vi "EVM_Sweep_Only_R_S_CMP180_SpecialCASE.vi"() -> ()   [LabVIEW 2023, in "EVM.lvlib"]
uses:
  lib/CTL/LitePoint_EVM_SG.ctl
  lib/CTL/LitePoint_EVM_SA.ctl
  EVM.lvlib
  lib/LitePoints/LitePoints.lvlib
  lib/FTDI/JIO/CLC_JIO_FTDI.lvlib
  lib/R_S/R_S.lvlib
panel:
  out "ReceivedPower":dbl format="%#.3g"
  out "Best EVM ALL":dbl
  out "PST(sec)":dbl
  out "Best EVM":dbl
  out "error out":errorcluster
  in  "Power res":i32=2
  in  "Stop Power":i32
  in  "Start Power":i32=-40
  in  "BFIC_ele_stop":i32=12
  in  "BFIC_ele_res":i32=4
  in  "BFIC_ele_start":i32
  in  "BFIC_com_stop":i32=12
  in  "BFIC_com_res":i32=4
  in  "BFIC_com_start":i32
  in  "UD_att_stop":i32=120
  in  "UD_att_res":i32=8
  in  "UD_att_start":i32
  out "UD_att":i32=255
  out "BFIC_com_step":i32=15
  out "BFIC_ele_step":i32=15
  out "SG Power":i32=-10
  in  "TRXmode":u16(ring)=1 items=["Tx"=1, "Rx"=2]
  in  "Polarity":u16(ring) items=["H", "V"]
  out "floder Exist?":bool=TRUE
  in  "Waiting \nTime(ms)":u32=1
  in  "FileNote":string="test16_wayne_MCS11"
  in  "SG":refnum<visa-resource-name>="TCPIP0::192.168.200.50::hislip0::INSTR"
  in  "SA":refnum<visa-resource-name>="TCPIP0::192.168.200.50::hislip0::INSTR"
  out "Spectrum Data":cluster{"X":dbl, "Y":dbl}[](graph)
  # "TMYTEK_CLC_JIO_R&S_EVM_CMP180_StartMaxPOWER"
  # "`"
  # "12"
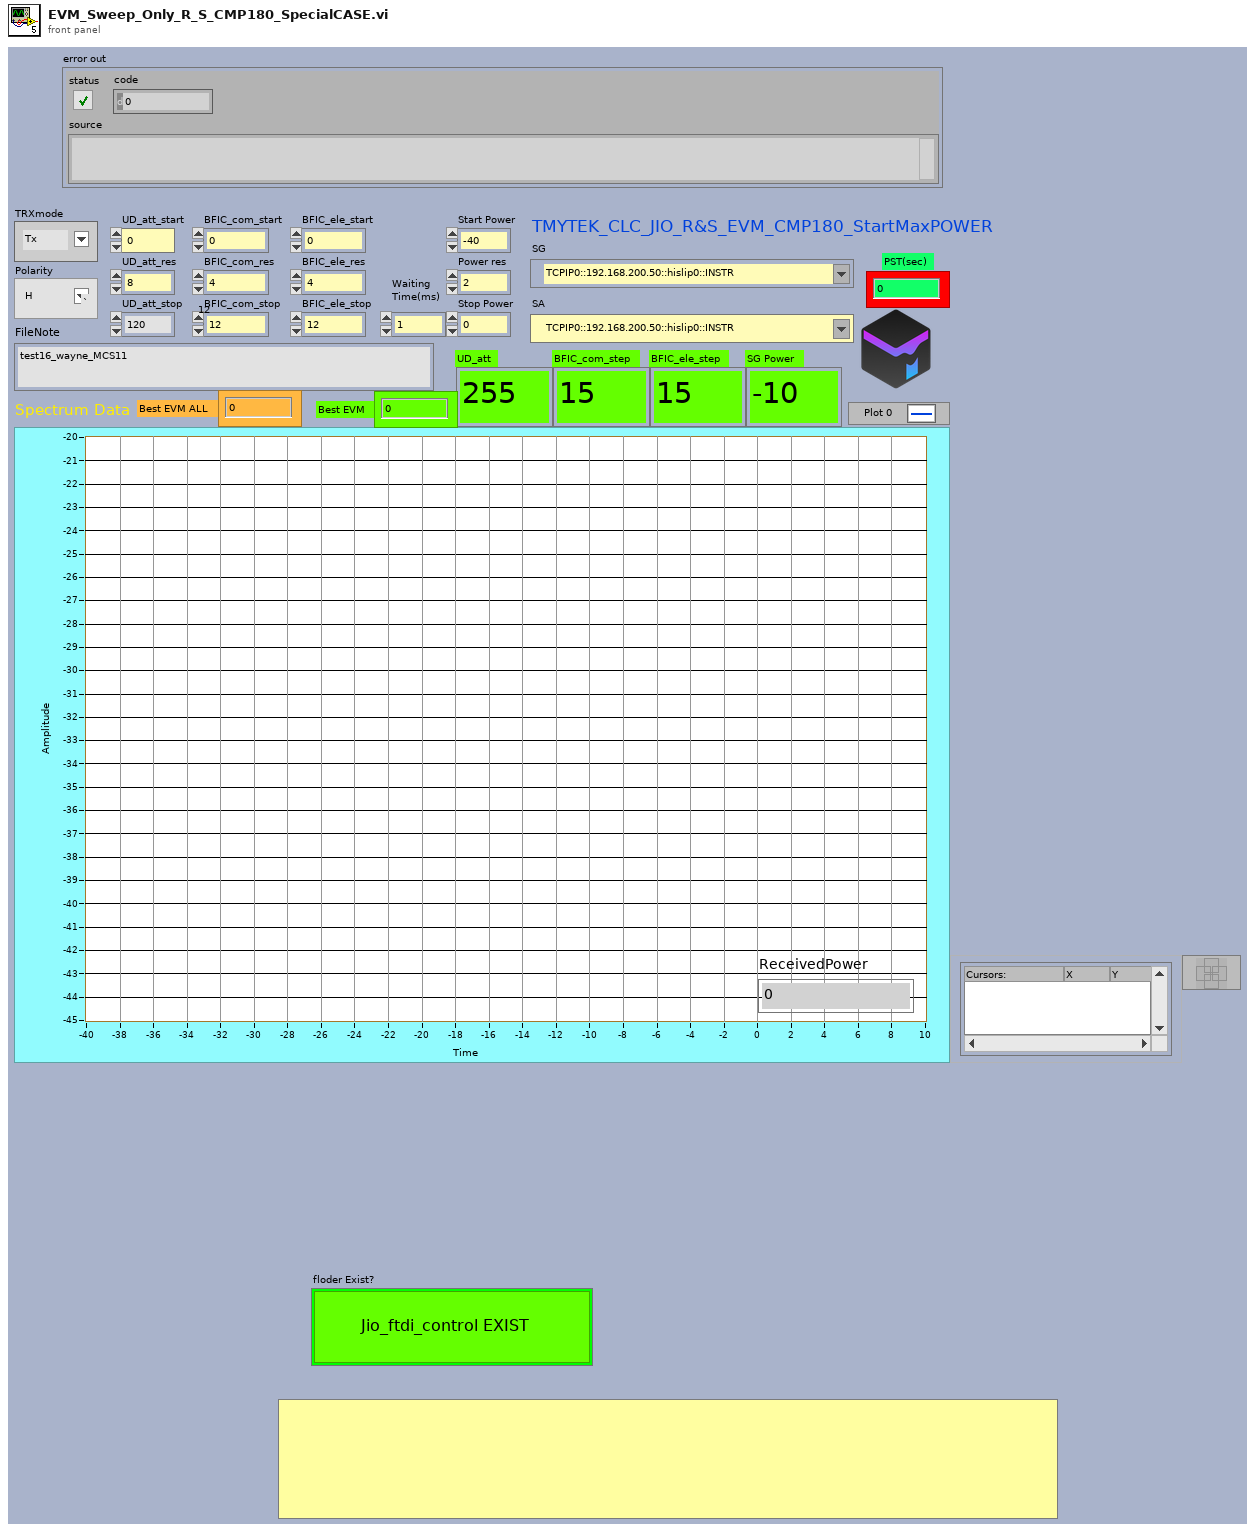
[diagram p1: front panel]
types:
  T1 = typedef "LitePoint_EVM_SG.ctl" = enum16{"Init", "Close", "set_SG", "AdjustLevel", "byPass", "RF_ON", "RF_OFF"}
  T2 = typedef "LitePoint_EVM_SA.ctl" = enum16{"Init", "Close", "set_SA", "get_EVM", "byPass", "getPower"}
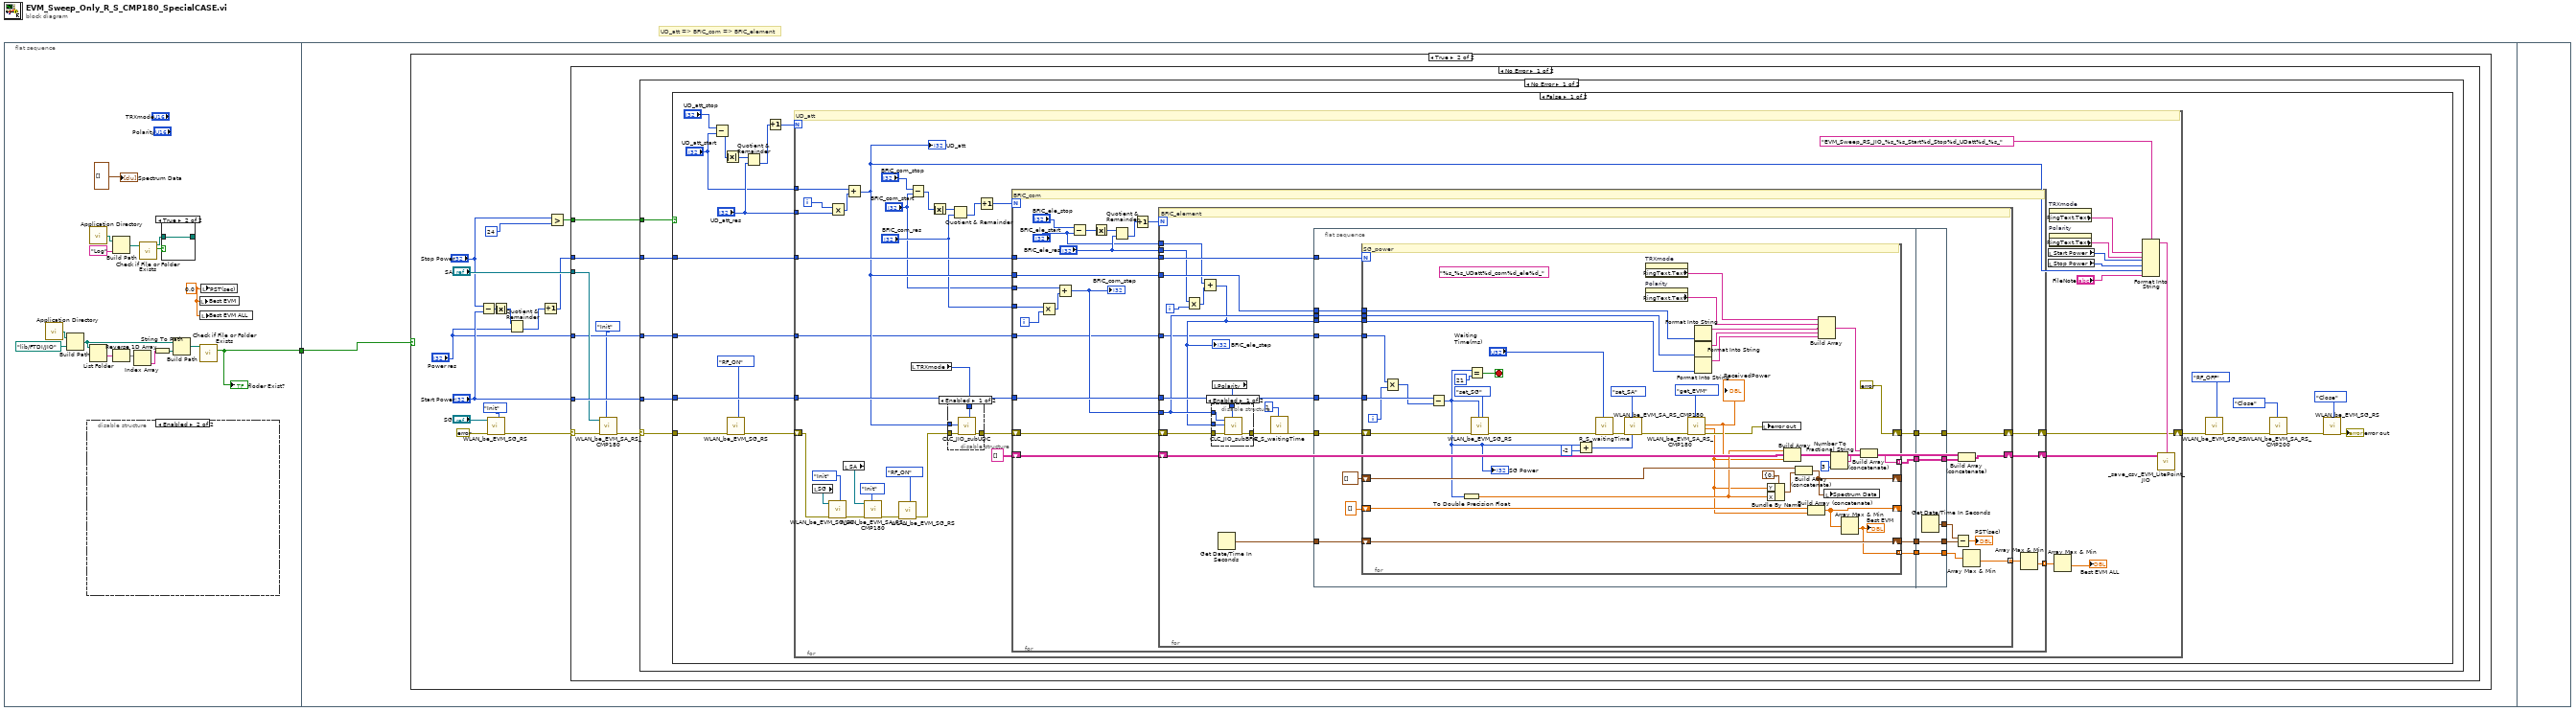
[diagram p0: block diagram]
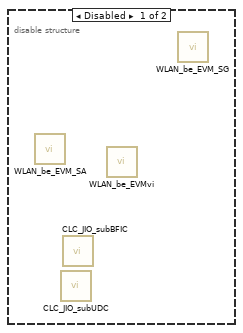
[diagram p2: hidden frame]
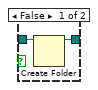
[diagram p3: hidden frame]
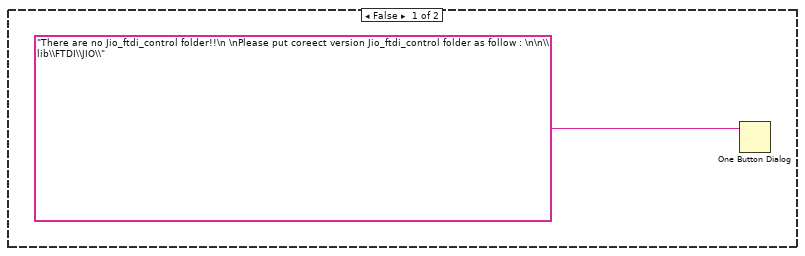
[diagram p4: hidden frame]
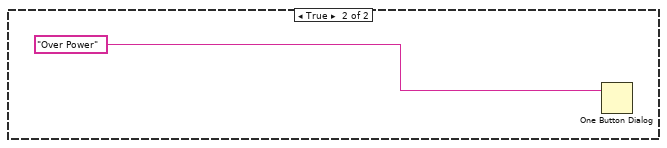
[diagram p7: hidden frame]
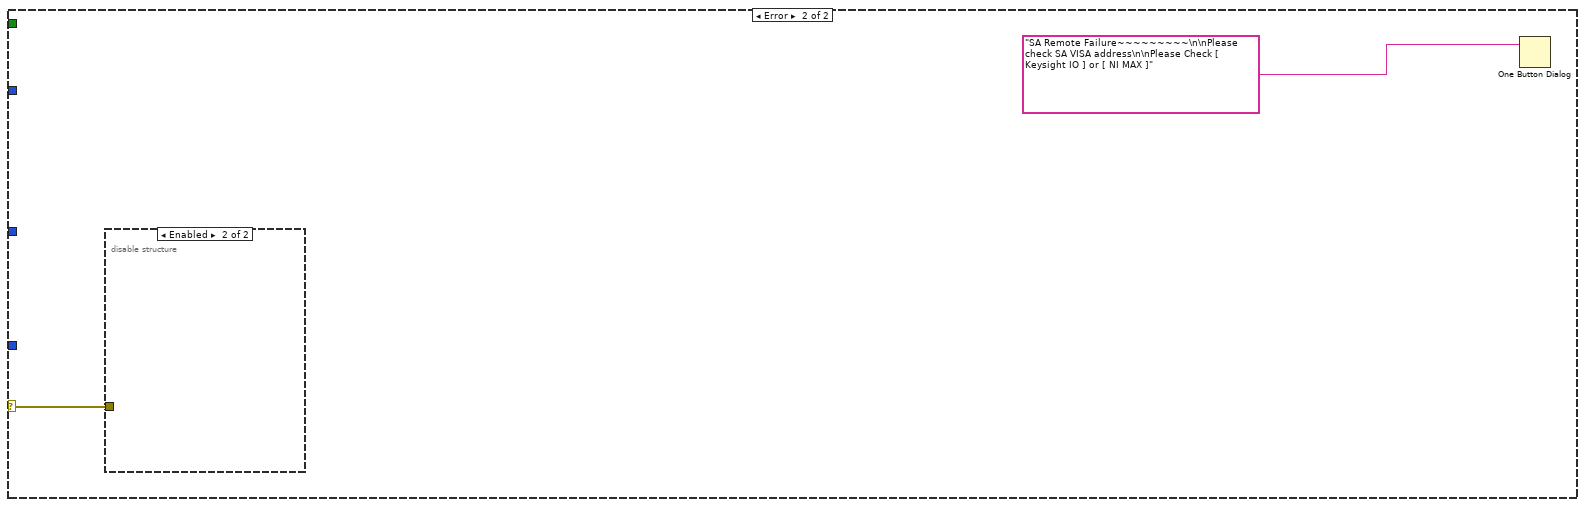
[diagram p8: hidden frame]
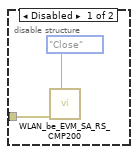
[diagram p9: hidden frame]
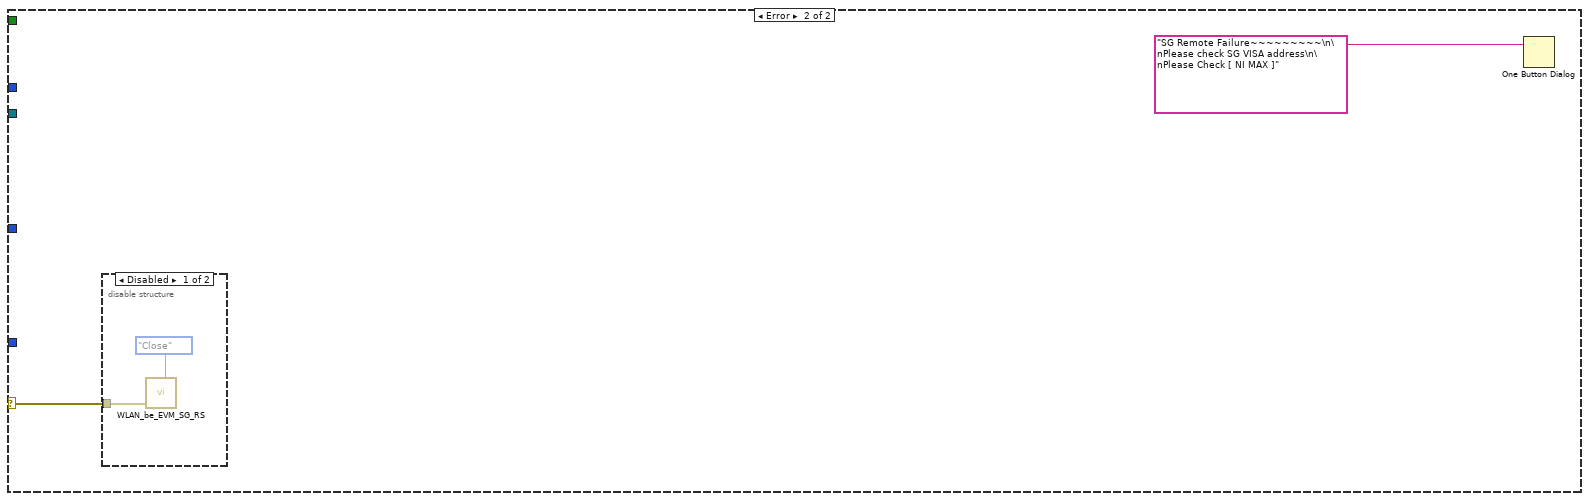
[diagram p10: hidden frame]
diagram:
  # "UD_att => BFIC_com => BFIC_element"
  n1 = flat-sequence {
    tunnel: [w3] -> w1
    tunnel: w1 -> [w21]
    frame #0 {
      w2 = 0.0 ("PST(sec)")
      n2 = call <vilib>:"Application Directory.vi"() -> ("Application Directory"=w9:path)
      n3 = Build Path(base path=w9, name or relative path=path "lib/FTDI/JIO") -> (appended path=w10:path)
      n4 = disable-structure shown="Enabled" {
        frame Disabled {
          n5 = call "WLAN_be_EVM_SA.vi"() -> ()  [unwired: 8 in, 4 out]
          n6 = call "CLC_JIO_subUDC.vi"() -> ()  [unwired: 10 in, 2 out]
          n7 = call "CLC_JIO_subBFIC.vi"() -> ()  [unwired: 10 in, 2 out]
          n8 = call "WLAN_be_EVMvi.vi"() -> ()  [unwired: 8 in, 4 out]
          n9 = call "WLAN_be_EVM_SG.vi"() -> ()  [unwired: 10 in, 2 out]
        }
        frame Enabled {
        }
      }
      n10 = call <vilib>:"Application Directory.vi"() -> ("Application Directory"=w16:path)
      n11 = List Folder(path=w10) -> (folder names=w5:string[])  [unwired: 3 in, 3 out]
      n12 = Reverse 1D Array(array=w5) -> (reversed array=w6:string[])
      n13 = Build Path(base path=w16, name or relative path="Log") -> (appended path=w13:path)
      n14 = Index Array(array=w6) -> (element=w7:string)  [unwired: 1 in]
      n15 = call <vilib>:"Check if File or Folder Exists.vi"("path"=w13) -> ("file or folder exists?"=w15:bool, "dup path"=w14:path)  [unwired: 8 in, 1 out]
      n16 = String To Path(string=w7) -> (path=w8:path)
      n17 = case shown="True" w15 {
        tunnel: w14 -> [w19 w20]
        tunnel: [w18 w20] -> _
        frame False {
          n18 = Create Folder(path (use dialog)=w19) -> (created path=w18:path)  [unwired: 2 in, 2 out]
        }
        frame True {
        }
      }
      n19 = Build Path(base path=w10, name or relative path=w8) -> (appended path=w11:path)
      n20 = local write "Best EVM"(w2) -> ()
      n21 = local write "Best EVM ALL"(w2) -> ()
      n22 = call <vilib>:"Check if File or Folder Exists.vi"("path"=w11) -> ("file or folder exists?"=w3:bool)  [unwired: 8 in, 2 out]
      "floder Exist?" <- w3
      n23 = local write "PST(sec)"(w2) -> ()
      "Spectrum Data" <- cluster{"X":dbl, "Y":dbl}[] [] ("XY Graph")
    }
    frame #1 {
      n24 = case shown="True" w21 {
        frame False {
          n25 = One Button Dialog(message="There are no Jio_ftdi_control folder!!\n \nPlease put coreect version Jio_ftdi_control folder as follow : \n\n\\lib\\FTDI\\JIO\\") -> ()  [unwired: 1 in, 1 out]
        }
        frame True {
          n26 = Subtract(x="Stop Power", y="Start Power") -> (x-y=w27:i32)
          n27 = call "WLAN_be_EVM_SG_RS.vi"("Function_SG"=LitePoint_EVM_SG."Init", "error in"=errorcluster {"status"=FALSE, "code"=0, "source"=""} ("error in (no error)"), "VISA IN"="SG") -> ("error out"=w29:errorcluster)  [unwired: 7 in, 1 out]
          n28 = Absolute Value(x=w27) -> (abs(x)=w23:i32)
          n29 = Quotient & Remainder(x=w23, y="Power res") -> (floor(x/y)=w26:i32)  [unwired: 1 out]
          n30 = Increment(x=w26) -> (x+1=w33:i32)
          n31 = Greater?(x="Stop Power", y=24) -> (0:w35:bool)
          n32 = case shown="No Error" w29 {
            selector: w29 -> [w41 w237]
            tunnel: "SA" -> [w39 _]
            tunnel: w35 -> [w44 _]
            tunnel: "Start Power" -> [w43 _]
            tunnel: w33 -> [w42 _]
            tunnel: "Power res" -> [w38 _]
            frame No Error {
              n33 = call "WLAN_be_EVM_SA_RS_CMP180.vi"("Function"=LitePoint_EVM_SA."Init", "error in"=w41, "VISA IN"=w39) -> ("error out"=w40:errorcluster)  [unwired: 4 in, 4 out]
              n34 = case shown="No Error" w40 {
                selector: w40 -> [w46 w233]
                tunnel: w44 -> [w49 _]
                tunnel: w43 -> [w48 _]
                tunnel: w42 -> [w47 _]
                tunnel: w38 -> [w45 _]
                frame No Error {
                  n35 = case shown="False" w49 {
                    tunnel: w48 -> [w68 _]
                    tunnel: w46 -> [w67 _]
                    tunnel: w47 -> [w69 _]
                    tunnel: w45 -> [w55 _]
                    frame False {
                      n36 = Subtract(x="UD_att_stop", y="UD_att_start") -> (x-y=w62:i32)
                      n37 = Absolute Value(x=w62) -> (abs(x)=w59:i32)
                      n38 = call "WLAN_be_EVM_SG_RS.vi"("Function_SG"=LitePoint_EVM_SG."RF_ON", "error in"=w67) -> ("error out"=w65:errorcluster)  [unwired: 8 in, 1 out]
                      n39 = Quotient & Remainder(x=w59, y="UD_att_res") -> (floor(x/y)=w60:i32)  [unwired: 1 out]
                      n40 = Increment(x=w60) -> (x+1=w56:i32)
                      n41 = for {
                        N: w56 -> [_]
                        tunnel: w69 -> [w107]
                        tunnel: w68 -> [w106]
                        shift-right: [w94] -> w64
                        shift-left: w65 -> [w79]
                        tunnel: "UD_att_res" -> [w91]
                        tunnel: "UD_att_start" -> [w90]
                        tunnel: w55 -> [w81]
                        i -> [w93]
                        # "UD_att"
                        n42 = local read "SG"() -> (w76:refnum<visa-resource-name>)
                        n43 = call "WLAN_be_EVM_SG_RS.vi"("Function_SG"=LitePoint_EVM_SG."Init", "error in"=w79, "VISA IN"=w76) -> ("error out"=w77:errorcluster)  [unwired: 7 in, 1 out]
                        n44 = Multiply(x=w93, y=w91) -> (x*y=w92:i32)
                        n45 = local read "SA"() -> (w75:refnum<visa-resource-name>)
                        n46 = Add(x=w90, y=w92) -> (x+y=w89:i32)
                        "UD_att" <- w89
                        n47 = call "WLAN_be_EVM_SA_RS_CMP180.vi"("Function"=LitePoint_EVM_SA."Init", "error in"=w77, "VISA IN"=w75) -> ("error out"=w73:errorcluster)  [unwired: 4 in, 4 out]
                        n48 = call "WLAN_be_EVM_SG_RS.vi"("Function_SG"=LitePoint_EVM_SG."RF_ON", "error in"=w73) -> ("error out"=w72:errorcluster)  [unwired: 8 in, 1 out]
                        n49 = Subtract(x="BFIC_com_stop", y="BFIC_com_start") -> (x-y=w88:i32)
                        n50 = local read "TRXmode"() -> (w103:u16)
                        n51 = Absolute Value(x=w88) -> (abs(x)=w87:i32)
                        n52 = disable-structure shown="Enabled" {
                          disable-tunnel: [w111 w112] -> w105
                          disable-tunnel: w72 -> [w110 w112]
                          disable-tunnel: w103 -> [w109 _]
                          disable-tunnel: w89 -> [w108 _]
                          frame Enabled {
                            n53 = call "CLC_JIO_subUDC.vi"("Mode"=w109, "error in"=w110, "ud att"=w108) -> ("error out"=w111:errorcluster)  [unwired: 7 in, 1 out]
                          }
                          frame Disabled {
                          }
                        }
                        n54 = Quotient & Remainder(x=w87, y="BFIC_com_res") -> (floor(x/y)=w83:i32)  [unwired: 1 out]
                        n55 = Increment(x=w83) -> (x+1=w82:i32)
                        n56 = for {
                          N: w82 -> [_]
                          tunnel: w107 -> [w134]
                          tunnel: w106 -> [w133]
                          shift-right: [w130] -> w104
                          shift-left: string[][] [] -> [w131]
                          tunnel: w89 -> [w129]
                          shift-right: [w128] -> w94
                          shift-left: w105 -> [w132]
                          tunnel: "BFIC_com_res" -> [w124]
                          tunnel: "BFIC_com_start" -> [w123]
                          tunnel: w81 -> [w115]
                          tunnel: [w113] -> w71 mode=indexing
                          i -> [w126]
                          # "BFIC_com"
                          n57 = Multiply(x=w124, y=w126) -> (x*y=w127:i32)
                          n58 = Add(x=w123, y=w127) -> (x+y=w125:i32)
                          "BFIC_com_step" <- w125
                          n59 = Subtract(x="BFIC_ele_stop", y="BFIC_ele_start") -> (x-y=w121:i32)
                          n60 = Absolute Value(x=w121) -> (abs(x)=w122:i32)
                          n61 = Quotient & Remainder(x=w122, y="BFIC_ele_res") -> (floor(x/y)=w119:i32)  [unwired: 1 out]
                          n62 = Increment(x=w119) -> (x+1=w116:i32)
                          n63 = for {
                            N: w116 -> [_]
                            tunnel: w134 -> [w163]
                            tunnel: w133 -> [w162]
                            shift-right: [w160] -> w130
                            shift-left: w131 -> [w159]
                            tunnel: w125 -> [w154]
                            tunnel: w129 -> [w155]
                            shift-right: [w138] -> w128
                            shift-left: w132 -> [w158]
                            tunnel: "BFIC_ele_res" -> [w149]
                            tunnel: "BFIC_ele_start" -> [w148]
                            tunnel: w115 -> [w147]
                            tunnel: [w135] -> w114 mode=indexing
                            i -> [w150]
                            # "BFIC_element"
                            n64 = Multiply(x=w149, y=w150) -> (x*y=w152:i32)
                            n65 = Add(x=w148, y=w152) -> (x+y=w151:i32)
                            "BFIC_ele_step" <- w151
                            n66 = local read "Polarity"() -> (w153:u16)
                            n67 = disable-structure shown="Enabled" {
                              disable-tunnel: w158 -> [w230 w231]
                              disable-tunnel: [w229 w231] -> w157
                              disable-tunnel: w151 -> [w228 _]
                              disable-tunnel: w154 -> [w227 _]
                              disable-tunnel: w153 -> [w226 _]
                              frame Enabled {
                                n68 = call "CLC_JIO_subBFIC.vi"("pol"=w226, "error in"=w230, "ele"=w228, "com"=w227) -> ("error out"=w229:errorcluster)  [unwired: 6 in, 1 out]
                              }
                              frame Disabled {
                              }
                            }
                            n69 = Get Date/Time In Seconds() -> (seconds since 1Jan1904=w145:timestamp)
                            n70 = call "R_S_waitingTime.vi"("Waiting Time(ms)"=u32 1, "error in"=w157) -> ("error out"=w146:errorcluster)  [unwired: 9 in]
                            n71 = flat-sequence {
                              tunnel: w163 -> [w177]
                              tunnel: w162 -> [w175]
                              tunnel: w155 -> [w173]
                              tunnel: w154 -> [w172]
                              tunnel: w151 -> [w170]
                              tunnel: w147 -> [w169]
                              tunnel: w146 -> [w168]
                              tunnel: w145 -> [w166]
                              tunnel: [w174] -> w143
                              tunnel: [w171] -> w142
                              tunnel: [w165] -> w141
                              tunnel: [w164] -> w137
                              tunnel: [w223] -> w144
                              tunnel: [w224] -> w138
                              tunnel: [w225] -> w161
                              tunnel: w143 -> [w225]
                              tunnel: w142 -> [w224]
                              tunnel: w141 -> [w223]
                              tunnel: [w222] -> w140
                              tunnel: [w221] -> w136
                              tunnel: w137 -> [w221]
                              frame #0 {
                                n72 = for {
                                N: w177 -> [_]
                                tunnel: w175 -> [w220]
                                shift-right: [errorcluster {"status"=FALSE, "code"=0, "source"=""} ("error out")] -> w171
                                shift-left: w168 -> [w212]
                                shift-right: [w214] -> _
                                shift-left: cluster{"X":dbl, "Y":dbl}[] [] ("XY Graph") -> [w216]
                                tunnel: [w204] -> w174 mode=indexing
                                tunnel: w173 -> [w201]
                                tunnel: w170 -> [w199]
                                tunnel: w172 -> [w200]
                                tunnel: w169 -> [w193]
                                shift-right: [w181] -> _
                                shift-left: dbl[] [] -> [w183]
                                shift-right: [w180] -> w165
                                shift-left: w166 -> [w180]
                                tunnel: [w178] -> w164 mode=indexing
                                i -> [w194]
                                stop <- w218 stop-if-true
                                (unwired) "%s_%s_UDatt%d_com%d_ele%d_" ("format string")
                                # "SG_power"
                                n73 = Multiply(x=w193, y=w194) -> (x*y=w192:i32)
                                n74 = Subtract(x=w220, y=w192) -> (x-y=w186:i32)
                                "SG Power" <- w186
                                n75 = To Double Precision Float(number=w186) -> (double precision float=w213:dbl)
                                n76 = Equal?(x=w186, y=21) -> (x = y?=w218:bool)
                                n77 = call "WLAN_be_EVM_SG_RS.vi"("Function_SG"=LitePoint_EVM_SG."set_SG", "setPower"=w186, "error in"=w212) -> ("error out"=w190:errorcluster)  [unwired: 7 in, 1 out]
                                n78 = Add(x=w186, y=-2) -> (x+y=w185:i32)
                                n79 = call "R_S_waitingTime.vi"("Waiting Time(ms)"="Waiting \nTime(ms)", "error in"=w190) -> ("error out"=w208:errorcluster)  [unwired: 9 in]
                                n80 = call "WLAN_be_EVM_SA_RS_CMP180.vi"("SG Power"=w185, "Function"=LitePoint_EVM_SA."set_SA", "error in"=w208) -> ("error out"=w188:errorcluster)  [unwired: 4 in, 4 out]
                                n81 = property on="TRXmode" class="Ring (strict)"() -> ("RingText.Text"=w203:string)  [unwired: 2 in, 2 out]
                                n82 = property on="Polarity" class="Ring (strict)"() -> ("RingText.Text"=w202:string)  [unwired: 2 in, 2 out]
                                n83 = call "WLAN_be_EVM_SA_RS_CMP180.vi"("Function"=LitePoint_EVM_SA."get_EVM", "error in"=w188) -> ("error out"=w187:errorcluster, "EVM"=w182:dbl, "Power"=w191:dbl)  [unwired: 5 in, 2 out]
                                "ReceivedPower" <- w191
                                n84 = Format Into String(w201) -> (resulting string=w198:string)  [unwired: 3 in, 1 out]
                                n85 = Format Into String(w200) -> (resulting string=w197:string)  [unwired: 3 in, 1 out]
                                n86 = Format Into String(w199) -> (resulting string=w196:string)  [unwired: 3 in, 1 out]
                                n87 = local write "error out"(w187) -> ()
                                n88 = Bundle By Name(cluster=cluster{"X":dbl, "Y":dbl} {"X"=0.0, "Y"=0.0} ("element"), "Y"=w182, "X"=w213) -> (w215:cluster{"X":dbl, "Y":dbl})
                                n89 = Build Array(w213, w191, w182) -> (w206:dbl[])
                                n90 = Build Array (concatenate)(w216, w215) -> (w214:cluster{"X":dbl, "Y":dbl}[])
                                n91 = Build Array (concatenate)(w183, w182) -> (w181:dbl[])
                                n92 = Build Array(w203, w202, w198, w197, w196) -> (w195:string[])
                                n93 = local write "Spectrum Data"(w214) -> ()
                                n94 = Number To Fractional String(number=w206, precision (6)=i16 3) -> (F-format string=w205:string[])  [unwired: 2 in]
                                n95 = Array Max & Min(array=w181) -> (min value=w178:dbl)  [unwired: 3 out]
                                "Best EVM" <- w178
                                n96 = Build Array (concatenate)(w195, w205) -> (w204:string[])
                                }
                              }
                              frame #1 {
                                n97 = Get Date/Time In Seconds() -> (seconds since 1Jan1904=w222:timestamp)
                              }
                            }
                            n98 = Subtract(x=w140, y=w144) -> (x-y=→"PST(sec)":dbl)
                            n99 = Build Array (concatenate)(w159, w161) -> (w160:string[][])
                            n100 = Array Max & Min(array=w136) -> (min value=w135:dbl)  [unwired: 3 out]
                          }
                          n101 = Array Max & Min(array=w114) -> (min value=w113:dbl)  [unwired: 3 out]
                        }
                        n102 = local read "Start Power"() -> (w98:i32)
                        n103 = local read "Stop Power"() -> (w100:i32)
                        n104 = property on="TRXmode" class="Ring (strict)"() -> ("RingText.Text"=w96:string)  [unwired: 2 in, 2 out]
                        n105 = property on="Polarity" class="Ring (strict)"() -> ("RingText.Text"=w97:string)  [unwired: 2 in, 2 out]
                        n106 = Array Max & Min(array=w71) -> (min value=→"Best EVM ALL":dbl)  [unwired: 3 out]
                        n107 = Format Into String(format string="EVM_Sweep_RS_JIO_%s_%s_Start%d_Stop%d_UDatt%d_%s_" ("delimiter (\\t)"), w96, w97, w98, w100, w89, "FileNote") -> (resulting string=w101:string)  [unwired: 2 in, 1 out]
                        n108 = call "_save_csv_EVM_LitePoint_JIO.vi"("delimiter (\\t)"=w101, "array in"=w104) -> ()  [unwired: 9 in, 1 out]
                      }
                      n109 = call "WLAN_be_EVM_SG_RS.vi"("Function_SG"=LitePoint_EVM_SG."RF_OFF", "error in"=w64) -> ("error out"=w52:errorcluster)  [unwired: 8 in, 1 out]
                      n110 = call "WLAN_be_EVM_SA_RS_CMP200.vi"("Function"=LitePoint_EVM_SA."Close", "error in"=w52) -> ("error out"=w51:errorcluster)  [unwired: 6 in, 3 out]
                      n111 = call "WLAN_be_EVM_SG_RS.vi"("Function_SG"=LitePoint_EVM_SG."Close", "error in"=w51) -> ("error out"=→"error out":errorcluster)  [unwired: 8 in, 1 out]
                    }
                    frame True {
                      n112 = One Button Dialog(message="Over Power") -> ()  [unwired: 1 in, 1 out]
                    }
                  }
                }
                frame Error {
                  n113 = disable-structure shown="Enabled" {
                    disable-tunnel: w233 -> [w236 _]
                    frame Disabled {
                      n114 = call "WLAN_be_EVM_SA_RS_CMP200.vi"("Function"=LitePoint_EVM_SA."Close", "error in"=w236) -> ()  [unwired: 6 in, 4 out]
                    }
                    frame Enabled {
                    }
                  }
                  n115 = One Button Dialog(message="SA Remote Failure~~~~~~~~~\n\nPlease check SA VISA address\n\nPlease Check [ Keysight IO ] or [ NI MAX ]") -> ()  [unwired: 1 in, 1 out]
                }
              }
            }
            frame Error {
              n116 = disable-structure shown="Disabled" {
                disable-tunnel: w237 -> [w240 _]
                frame Disabled {
                  n117 = call "WLAN_be_EVM_SG_RS.vi"("Function_SG"=LitePoint_EVM_SG."Close", "error in"=w240) -> ()  [unwired: 8 in, 2 out]
                }
                frame Enabled {
                }
              }
              n118 = One Button Dialog(message="SG Remote Failure~~~~~~~~~\n\nPlease check SG VISA address\n\nPlease Check [ NI MAX ]") -> ()  [unwired: 1 in, 1 out]
            }
          }
        }
      }
    }
    frame #2 {
    }
  }
